vi "time_stamp.vi"(7 "time_stamp":bool, 11 "String in":string) -> (3 "String out":string)   [LabVIEW 2019]
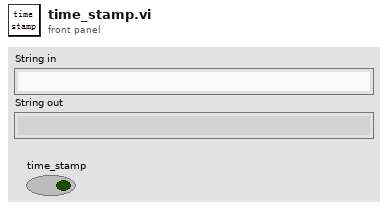
[diagram p1: front panel]
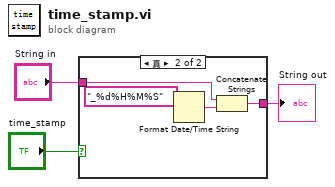
[diagram p0: block diagram]
diagram:
  n1 = case shown="真" "time_stamp" {
    tunnel: "String in" -> [w4 w6]
    tunnel: [w4 w5] -> w1
    frame False {
    }
    frame True {
      n2 = Format Date/Time String(time format string (%c)="_%d%H%M%S" ("时间格式字符串(%c)")) -> (date/time string=w8:string)  [unwired: 2 in]
      n3 = Concatenate Strings(w6, w8) -> (w5:string)
    }
  }
  "String out" <- w1
